vi "Motors Save.vi"(2 "error in":errorcluster, 3 "VISA in":refnum<visa-resource-name>="COM7") -> (0 "error out":errorcluster, 1 "VISA out":refnum<visa-resource-name>)   [LabVIEW 2018]
panel:
  in  "milliseconds to wait 4":u32
  in  "milliseconds to wait 3":u32
  in  "milliseconds to wait 2":u32
  in  "milliseconds to wait":u32
  out "BA 4":string
  out "BA 3":string
  out "BA 2":string
  out "BA 1":string
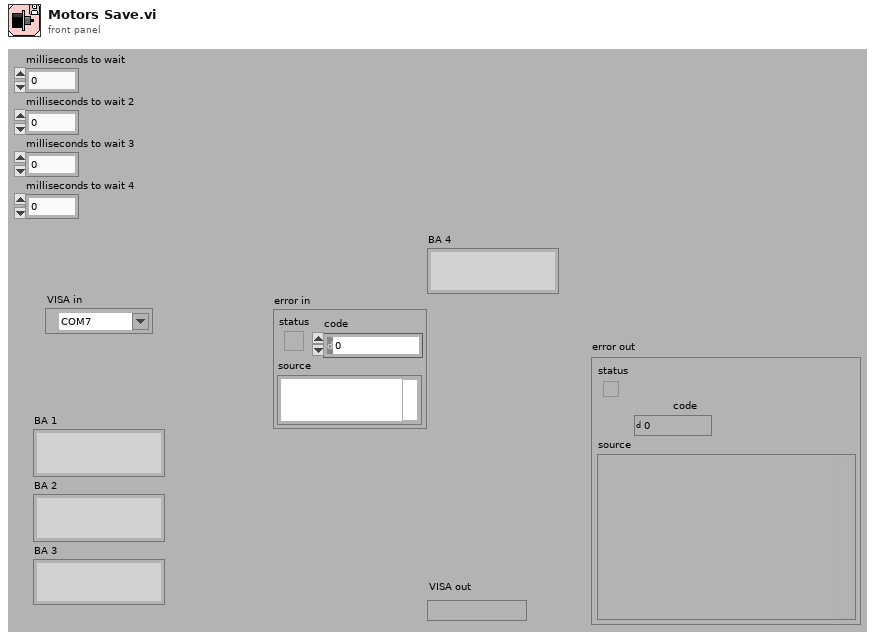
[diagram p1: front panel]
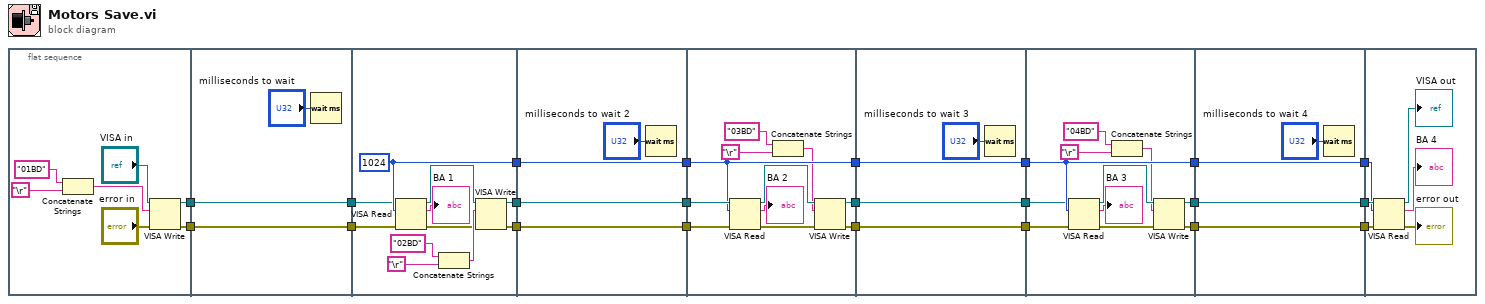
[diagram p0: block diagram]
diagram:
  n1 = flat-sequence {
    tunnel: [w26] -> w22
    tunnel: [w25] -> w21
    tunnel: w22 -> [w32]
    tunnel: w21 -> [w31]
    tunnel: [w32] -> w20
    tunnel: [w31] -> w19
    tunnel: w20 -> [w35]
    tunnel: w19 -> [w38]
    tunnel: [w33] -> w18
    tunnel: [w36] -> w17
    tunnel: [w39] -> w16
    tunnel: w18 -> [w47]
    tunnel: w17 -> [w46]
    tunnel: w16 -> [w45]
    tunnel: [w47] -> w15
    tunnel: [w46] -> w14
    tunnel: [w45] -> w13
    tunnel: w15 -> [w57]
    tunnel: w14 -> [w58]
    tunnel: w13 -> [w56]
    tunnel: [w56] -> w12
    tunnel: [w49] -> w10
    tunnel: [w48] -> w8
    tunnel: w12 -> [w62]
    tunnel: [w62] -> w11
    tunnel: w10 -> [w60]
    tunnel: [w60] -> w9
    tunnel: w8 -> [w59]
    tunnel: [w59] -> w7
    tunnel: w11 -> [w73]
    tunnel: w9 -> [w72]
    tunnel: w7 -> [w71]
    tunnel: [w73] -> w6
    tunnel: [w64] -> w3
    tunnel: [w63] -> w1
    tunnel: w6 -> [w77]
    tunnel: [w77] -> w5
    tunnel: [w75] -> w4
    tunnel: w3 -> [w75]
    tunnel: [w74] -> w2
    tunnel: w1 -> [w74]
    tunnel: w5 -> [w78]
    tunnel: w4 -> [w80]
    tunnel: w2 -> [w79]
    frame #0 {
      n2 = Concatenate Strings("01BD" ("Initial command 1"), "\r") -> (w27:string)
      n3 = VISA Write(VISA resource name="VISA in", write buffer=w27, error in (no error)="error in") -> (VISA resource name out=w25:refnum<visa-resource-name>, error out=w26:errorcluster)  [unwired: 1 out]
    }
    frame #1 {
      n4 = Wait (ms)(milliseconds to wait="milliseconds to wait") -> ()  [unwired: 1 out]
    }
    frame #2 {
      w39 = u32 1024 ("byte count")
      n5 = VISA Read(VISA resource name=w38, byte count=w39, error in (no error)=w35) -> (VISA resource name out=w37:refnum<visa-resource-name>, read buffer=→"BA 1":string, error out=w34:errorcluster)  [unwired: 1 out]
      n6 = Concatenate Strings("02BD" ("Initial command 2"), "\r") -> (w40:string)
      n7 = VISA Write(VISA resource name=w37, write buffer=w40, error in (no error)=w34) -> (VISA resource name out=w36:refnum<visa-resource-name>, error out=w33:errorcluster)  [unwired: 1 out]
    }
    frame #3 {
      n8 = Wait (ms)(milliseconds to wait="milliseconds to wait 2") -> ()  [unwired: 1 out]
    }
    frame #4 {
      n9 = VISA Read(VISA resource name=w58, byte count=w56, error in (no error)=w57) -> (VISA resource name out=w54:refnum<visa-resource-name>, read buffer=→"BA 2":string, error out=w53:errorcluster)  [unwired: 1 out]
      n10 = Concatenate Strings("03BD" ("Initial command 3"), "\r") -> (w50:string)
      n11 = VISA Write(VISA resource name=w54, write buffer=w50, error in (no error)=w53) -> (VISA resource name out=w49:refnum<visa-resource-name>, error out=w48:errorcluster)  [unwired: 1 out]
    }
    frame #5 {
      n12 = Wait (ms)(milliseconds to wait="milliseconds to wait 3") -> ()  [unwired: 1 out]
    }
    frame #6 {
      n13 = VISA Read(VISA resource name=w72, byte count=w73, error in (no error)=w71) -> (VISA resource name out=w69:refnum<visa-resource-name>, read buffer=→"BA 3":string, error out=w68:errorcluster)  [unwired: 1 out]
      n14 = Concatenate Strings("04BD" ("Initial command 4"), "\r") -> (w65:string)
      n15 = VISA Write(VISA resource name=w69, write buffer=w65, error in (no error)=w68) -> (VISA resource name out=w64:refnum<visa-resource-name>, error out=w63:errorcluster)  [unwired: 1 out]
    }
    frame #7 {
      n16 = Wait (ms)(milliseconds to wait="milliseconds to wait 4") -> ()  [unwired: 1 out]
    }
    frame #8 {
      n17 = VISA Read(VISA resource name=w80, byte count=w78, error in (no error)=w79) -> (VISA resource name out=→"VISA out":refnum<visa-resource-name>, read buffer=→"BA 4":string, error out=→"error out":errorcluster)  [unwired: 1 out]
    }
  }
